vi "FRIC_navX_Internal_Serial_ProcessingLoop.vi"(7 "Device Number":T3, 11 "Rate (4Hz-200Hz)":u8=50 min=4 max=200) -> ()   [LabVIEW 2016, in "navX Library.lvlib"]
doc: "This navX VI handles the reading/writing for the navX. All of the good stuff is in here.\nTHIS VI SHOULD NOT BE CALLED BY THE USER!"
uses:
  navX Library.lvlib
  _TypeDefs/Z900_navX_SerialStreamTypeDef.ctl
  _TypeDefs/FRIC_navX_DeviceNumbersTypeDef.ctl
  <vilib>/Rock Robotics/WPI/SerialPort/WPI_SerialPort.ctl
  _TypeDefs/FRIC_navX_I2C Process Loop TypeDef.ctl
  _TypeDefs/FRIC_navX_ProcessingLoopStatesTypeDef_I2C.ctl
  _TypeDefs/Z900_navX_DeviceTypeDef.ctl
  _TypeDefs/Z900_navX_ProtocolTypeDef.ctl
  _TypeDefs/Z900_navX_NotifyPacketTypeDef.ctl
  _TypeDefs/Z900_navX_ActionTypeDef.ctl
  <vilib>/Rock Robotics/SystemInterfaces/i2clib/i2c_bus.ctl
  _TypeDefs/Z900_navX_IntegrationControlRegisters.ctl
  <vilib>/Rock Robotics/WPI/SPI/WPI_SPIDevRef.ctl
  <vilib>/Rock Robotics/SystemInterfaces/spilib/spi_bus.ctl
  <vilib>/Rock Robotics/WPI/SerialPort/WPI_SerialPortRef.ctl
  <vilib>/Platform/TimedLoop/XDataNode/timing_clust.ctl
  <vilib>/Platform/TimedLoop/XDataNode/nitl_modes.ctl
  <vilib>/Platform/TimedLoop/XDataNode/wakeup.ctl
  <vilib>/Rock Robotics/SystemInterfaces/Utilities/FPGA_UtilitiesRead LocalTime.vi
  <vilib>/Platform/TimedLoop/XDataNode/XDataNode.xnode
  <vilib>/Platform/TimedLoop/XDataNode/XDNodeRunTimeDep.lvlib
panel:
  in  "Tab Control":enum32{"Page 1", "Page 2"}(tab)
  in  "Halt":bool
  out "Connected":bool
  out "error":errorcluster
  in  "Stream Type":T1=enum."AHRSAndPositioning"
  in  "Serial Port":T2=enum."MXP TTL"
  out "Loop Time":i64
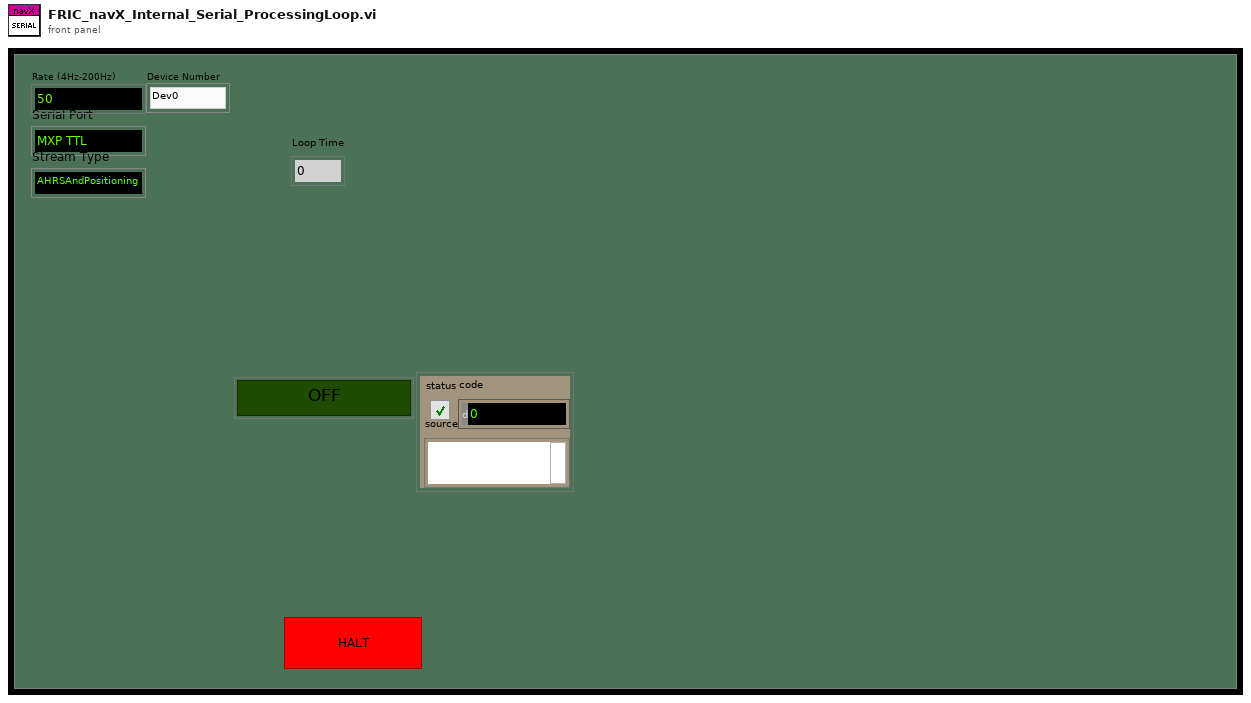
[diagram p1: front panel]
types:
  T1 = typedef "navX Library.lvlib/Z900_navX_SerialStreamTypeDef.ctl" = enum16{"YRPH", "Quaterinons", "Gyro/Raw", "AHRS", "AHRSAndPositioning", "AHRSAndPOSTime"}
  T2 = typedef "WPI_SerialPort.ctl" = enum16{"Onboard RS-232", "MXP TTL", "USB 1", "USB 2"}
  T3 = typedef "navX Library.lvlib/FRIC_navX_DeviceNumbersTypeDef.ctl" = enum16{"Dev0", "Dev1", "Dev2", "Dev3"}
  T4 = typedef "navX Library.lvlib/FRIC_navX_I2C Process Loop TypeDef.ctl" = cluster{"State Array":T5[], "error":errorcluster, "FPGA Cluster":cluster{"Last Valid FPGA Time":dbl, "Error Count":i32, "Initialized":bool}, "Device Info":T6, "I2CDevRef":cluster{"DevStatus":errorcluster, "Device Address":u8, "Handle":i32, "I2C Bus":T8}, "Registry":u8[], "Command Array":T9[], "Connected?":bool, "navX Device Memory Size":i32, "notification":T10, "Memory Size Set":bool, "SPIDevRef":T12, "navX Serial Open":cluster{"Stream Type":T1, "Serial Port":T2}, "SerialPortRef":T14, "Serial Read Buffer":string, "Serial Write Buffer":string[], "Device Number":T3, "navX SPI Open":cluster{"SPI Bus":T13, "Clock Rate (Hz)":dbl}, "Loop dt":i64, "current time":timestamp, "Loop Time":i64}
  T5 = typedef "navX Library.lvlib/FRIC_navX_ProcessingLoopStatesTypeDef_I2C.ctl" = enum16{"Process", "INI", "Check Packets Valid", "Close", "Clear VISA", "Generate Command", "Last Packet Valid", "Open", "Read", "Reset Serial", "Set Termination Char", "Update AE", "Wait", "Write", "Exit"}
  T6 = typedef "navX Library.lvlib/Z900_navX_DeviceTypeDef.ctl" = cluster{"Interface":cluster{"Protocol":T7, "Update Rate (4Hz-200Hz)":u8, "navX Open TypeDef":variant}, "Notify Packet":refnum<notifier>, "Loop VI Refnum":refnum<vi>, "Ready to Close Occurrence Refnum":refnum<k4>, "Name":string}
  T7 = typedef "navX Library.lvlib/Z900_navX_ProtocolTypeDef.ctl" = enum16{"SERIAL", "I2C", "SPI"}
  T8 = typedef "i2c_bus.ctl" = enum16{"I2C On-Board", "I2C MXP", "Invalid"}
  T9 = typedef "navX Library.lvlib/Z900_navX_IntegrationControlRegisters.ctl" = u8
  T10 = typedef "navX Library.lvlib/Z900_navX_NotifyPacketTypeDef.ctl" = cluster{"navX Action":T11, "Data":variant, "Stream Type":T1, "Device Number":T3}
  T11 = typedef "navX Library.lvlib/Z900_navX_ActionTypeDef.ctl" = enum16{"None", "Halt", "Normal Read", "Update Serial Protocol", "Update Rate Htz", "Zero-Yaw", "Zero-Displacement", "Zero-Velocity"}
  T12 = typedef "WPI_SPIDevRef.ctl" = cluster{"DevStatus":errorcluster, "Handle":i32, "SPI Bus":T13}
  T13 = typedef "spi_bus.ctl" = enum16{"SPI On-Board, CS0", "SPI On-Board, CS1", "SPI On-Board, CS2", "SPI On-Board, CS3", "SPI MXP", "Invalid"}
  T14 = typedef "WPI_SerialPortRef.ctl" = cluster{"DevStatus":errorcluster, "Serial Port Name":refnum<visa-resource-name>}
  T15 = typedef "XDNodeRunTimeDep.lvlib/timing_clust.ctl" = cluster{"Expected End [f-1]":u64, "Actual End [f-1]":u64, "Finished Late? [f-1]":bool, "Expected End [i-1]":u64, "Actual End [i-1]":u64, "Finished Late? [i-1]":bool, "Expected Start [i]":u64, "Actual Start [i]":u64, "Expected Start [f]":u64, "Actual Start [f]":u64, "Source Name":string, "Structure Name":string, "Period":i64, "Deadline":i64, "Offset":i64, "Start":i64, "Priority":i32, "Timeout":i32, "Mode":T16, "Wakeup Reason":T17, "Error":errorcluster, "Source Type":string, "Secondary Source Type":string, "Global End Time":u64, "Global Start Time":u64, "Frame Duration":u64, "Iteration Duration":u64, "Assigned CPU":i32, "I/O Scan Engine Mode":u32}
  T16 = typedef "XDNodeRunTimeDep.lvlib/nitl_modes.ctl" = enum32{"No Change", "Process missed periods, maintain original phase", "Discard missed periods, maintain original phase", "Process missed periods, ignore original phase", "Discard missed periods, ignore original phase"}
  T17 = typedef "XDNodeRunTimeDep.lvlib/wakeup.ctl" = enum32{"Normal", "Aborted", "Asynchronous wakeup", "Timing source error", "Timed loop error", "Timeout"}
  T18 = cluster{"Last Valid FPGA Time":dbl, "Error Count":i32, "Initialized":bool}
  T19 = typedef "Z900_navX_NotifyPacketTypeDef.ctl" = cluster{"navX Action":T20, "Data":variant, "Stream Type":T21, "Device Number":T22}
  T20 = typedef "Z900_navX_ActionTypeDef.ctl" = enum16{"None", "Halt", "Normal Read", "Update Serial Protocol", "Update Rate Htz", "Zero-Yaw", "Zero-Displacement", "Zero-Velocity"}
  T21 = typedef "Z900_navX_SerialStreamTypeDef.ctl" = enum16{"YRPH", "Quaterinons", "Gyro/Raw", "AHRS", "AHRSAndPositioning", "AHRSAndPOSTime"}
  T22 = typedef "FRIC_navX_DeviceNumbersTypeDef.ctl" = enum16{"Dev0", "Dev1", "Dev2", "Dev3"}
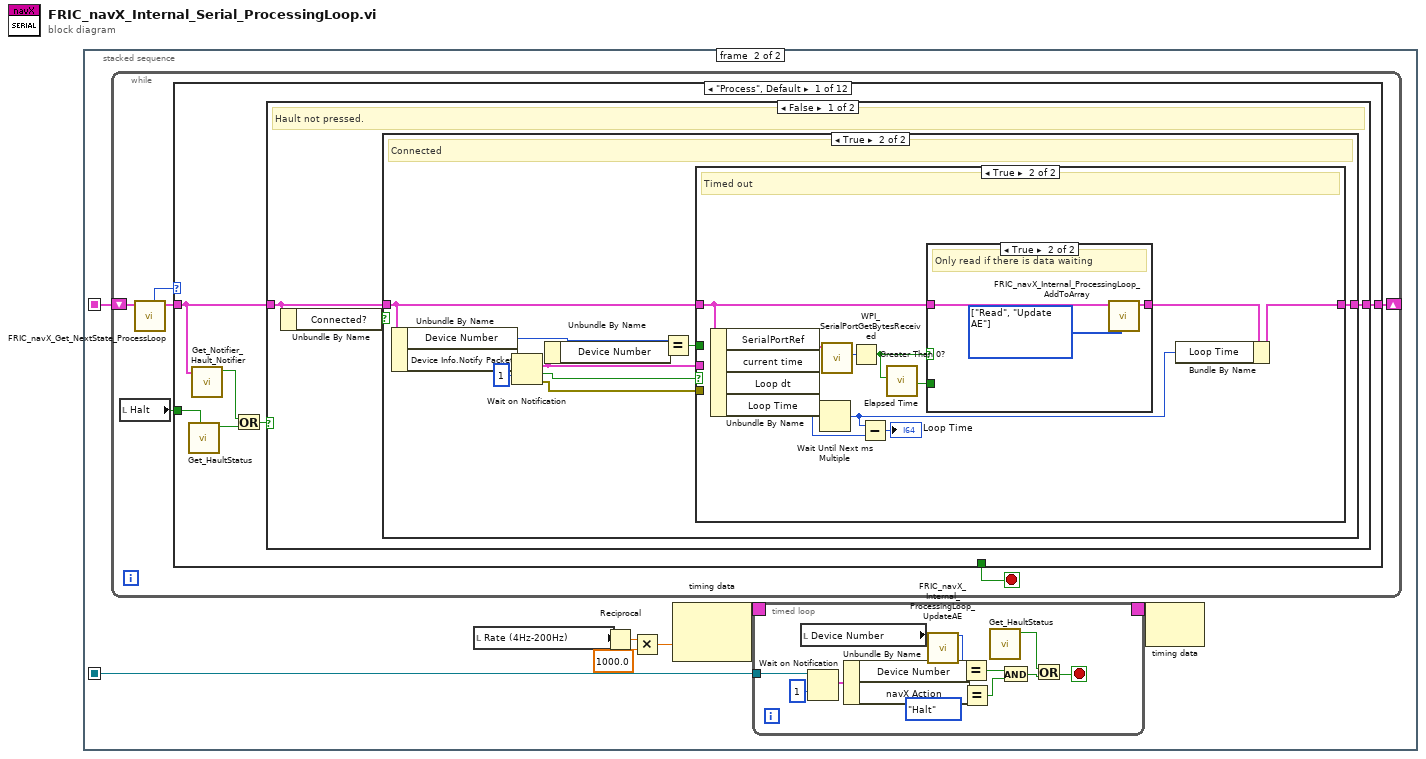
[diagram p0: block diagram]
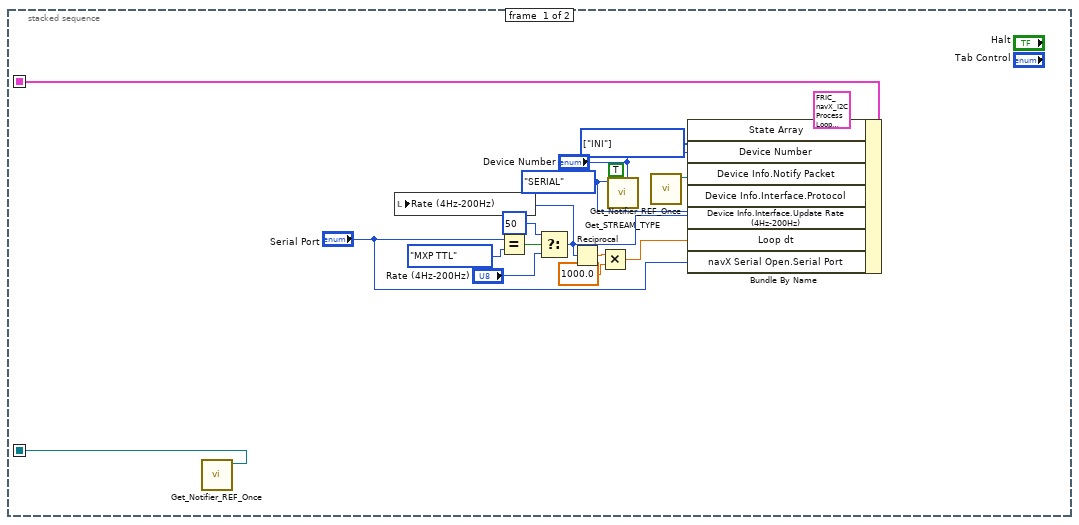
[diagram p2: hidden frame]
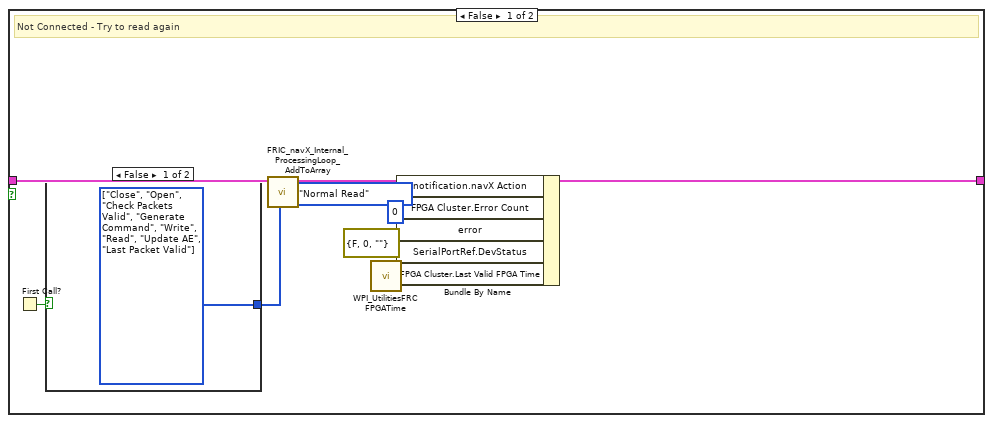
[diagram p3: hidden frame]
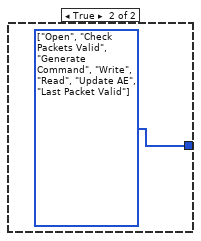
[diagram p4: hidden frame]
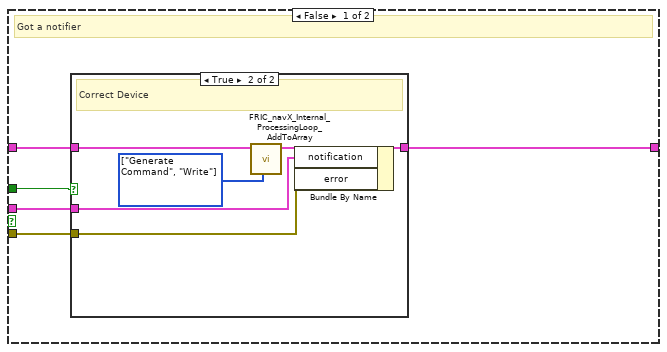
[diagram p5: hidden frame]
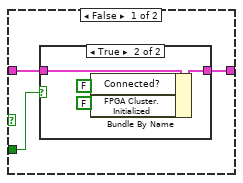
[diagram p7: hidden frame]
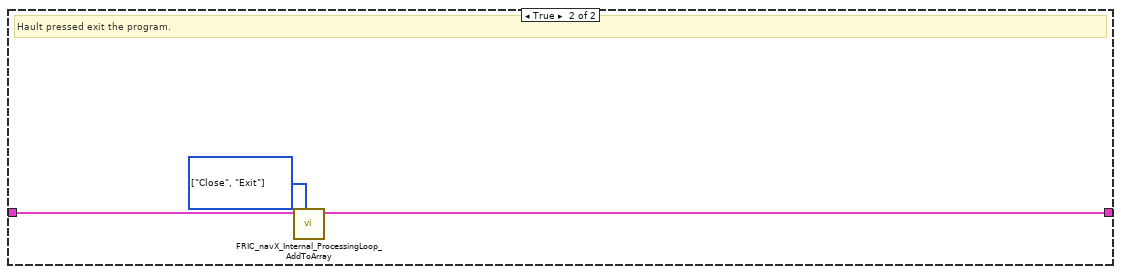
[diagram p9: hidden frame]
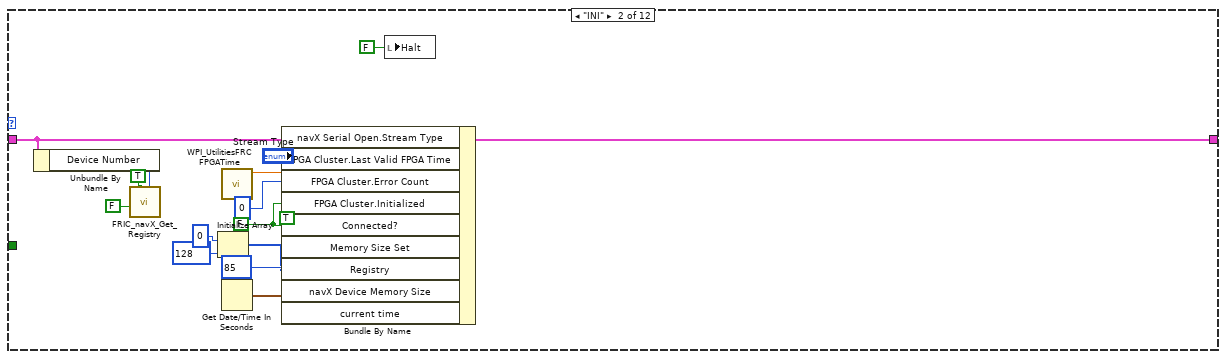
[diagram p10: hidden frame]
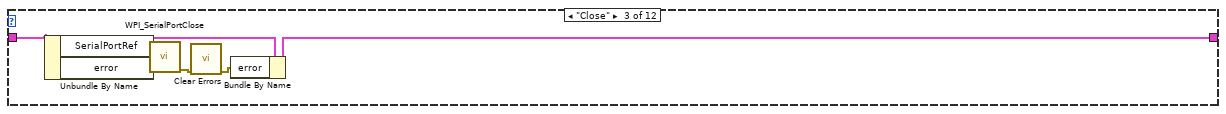
[diagram p11: hidden frame]
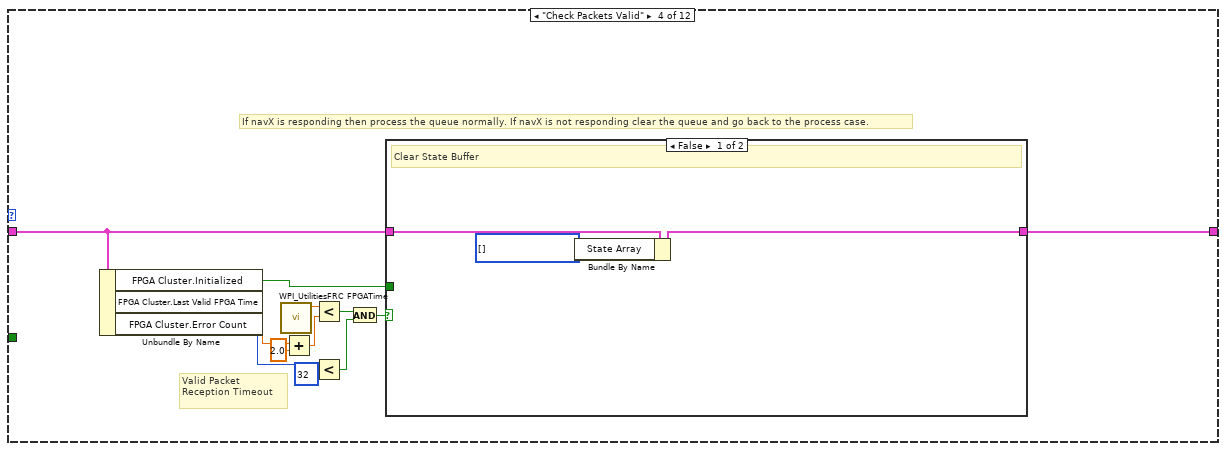
[diagram p12: hidden frame]
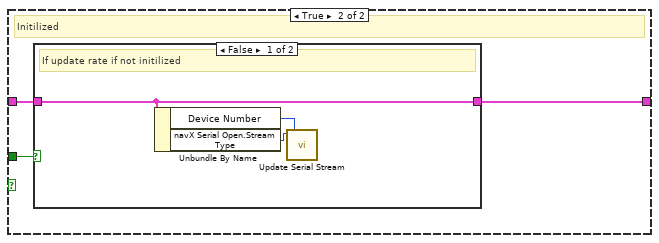
[diagram p13: hidden frame]
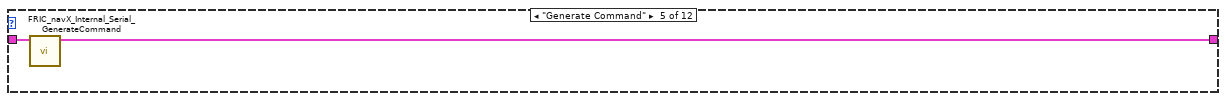
[diagram p15: hidden frame]
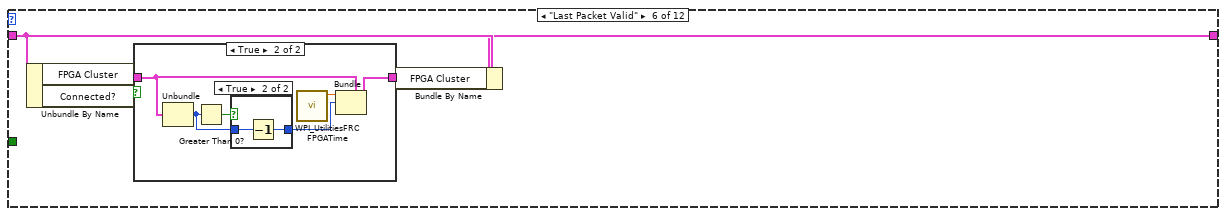
[diagram p16: hidden frame]
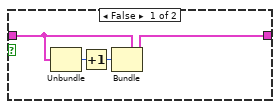
[diagram p17: hidden frame]
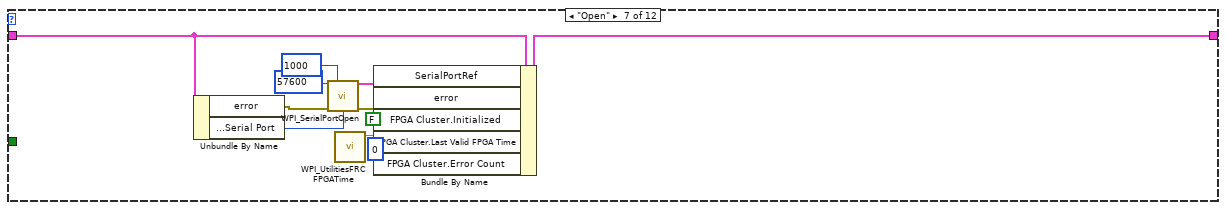
[diagram p19: hidden frame]
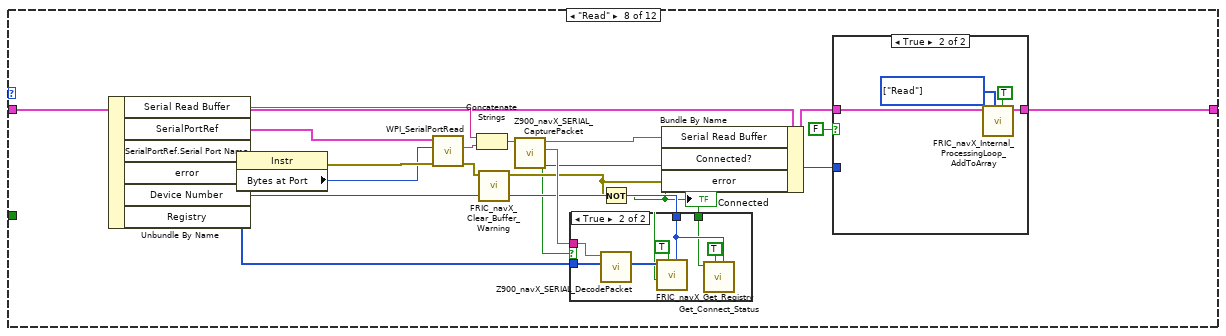
[diagram p20: hidden frame]
diagram:
  n1 = stacked-sequence {
    seq-local: [w17 _] -> [_ w25]
    seq-local: [w13 _] -> [_ w18]
    frame #0 {
      w1 = Z900_navX_ProtocolTypeDef."SERIAL" ("Protocol")
      w15 = T5[] [enum."INI"] items=["Process", "INI", "Check Packets Valid", "Close", "Clear VISA", "Generate Command", "Last Packet Valid", "Open", "Read", "Reset Serial", "Set Termination Char", "Update AE", "Wait", "Write", "Exit"] ("State Array")
      n2 = call "Get_Notifier_REF_Once.vi"() -> ("notifier ref out"=w13:refnum<notifier>)  [unwired: 10 in, 1 out]
      n3 = Equal?(x="Serial Port", y=WPI_SerialPort."MXP TTL") -> (x = y?=w11:bool)
      n4 = Select(t=u8 50, s=w11, f="Rate (4Hz-200Hz)") -> (s? t:f=w6:u8)
      n5 = local write "Rate (4Hz-200Hz)"(w6) -> ()
      n6 = Reciprocal(x=w6) -> (1/x=w9:dbl)
      n7 = Multiply(x=w9, y=1000.0) -> (x*y=w7:dbl)
      n8 = call "Get_STREAM_TYPE.vi"("Device Number"="Device Number", "Update"=TRUE, "Protocol (in)"=w1) -> ()  [unwired: 8 in, 1 out]
      n9 = call "Get_Notifier_REF_Once.vi"() -> ("notifier ref out"=w14:refnum<notifier>)  [unwired: 10 in, 1 out]
      n10 = Bundle By Name(cluster=T4 {"State Array"=[enum."INI", enum."Open"], "error"={"status"=FALSE, "code"=0, "source"=""}, "FPGA Cluster"={"Last Valid FPGA Time"=0.0, "Error Count"=0, "Initialized"=FALSE}, "Device Info"={"Interface"={"Protocol"=enum."SERIAL", "Update Rate (4Hz-200Hz)"=4, "navX Open TypeDef"=variant}, "Notify Packet"=refnum, "Loop VI Refnum"=refnum, "Ready to Close Occurrence Refnum"=refnum, "Name"=""}, "I2CDevRef"={"DevStatus"={"status"=FALSE, "code"=0, "source"=""}, "Device Address"=0, "Handle"=0, "I2C Bus"=enum."Invalid"}, "Registry"=[], "Command Array"=[214, 32], "Connected?"=FALSE, "navX Device Memory Size"=85, "notification"={"navX Action"=enum."None", "Data"=variant, "Stream Type"=enum."YRPH", "Device Number"=enum."Dev0"}, "Memory Size Set"=FALSE, "SPIDevRef"={"DevStatus"={"status"=FALSE, "code"=0, "source"=""}, "Handle"=0, "SPI Bus"=enum."SPI On-Board, CS0"}, "navX Serial Open"={"Stream Type"=enum."YRPH", "Serial Port"=enum."Onboard RS-232"}, "SerialPortRef"={"DevStatus"={"status"=FALSE, "code"=0, "source"=""}, "Serial Port Name"=""}, "Serial Read Buffer"="", "Serial Write Buffer"=[], "Device Number"=enum."Dev0", "navX SPI Open"={"SPI Bus"=enum."SPI MXP", "Clock Rate (Hz)"=500000.0}, "Loop dt"=0, "current time"=timestamp(0 s since 1904-01-01), "Loop Time"=0} ("I2C Process Loop TypeDef"), "State Array"=w15, "Device Number"="Device Number", "Device Info.Notify Packet"=w14, "Device Info.Interface.Protocol"=w1, "Device Info.Interface.Update Rate (4Hz-200Hz)"=w6, "Loop dt"=w7, "navX Serial Open.Serial Port"="Serial Port") -> (w17:T4)
    }
    frame #1 {
      n11 = while {
        shift-right: [w45] -> _
        shift-left: w25 -> [w48]
        stop <- w49 stop-if-true
        n12 = local read "Halt"() -> (w44:bool)
        n13 = call "FRIC_navX_Get_NextState_ProcessLoop.vi"("I2C Process Loop TypeDef (in)"=w48) -> ("I2C Process Loop TypeDef (out)"=w47:T4, "Current State"=w46:T5)  [unwired: 9 in]
        n14 = case shown="\"Process\", Default" w46 {
          tunnel: [_ _ _ _ _ _ _ _ _ _ TRUE _] -> w49
          tunnel: w47 -> [w53 w121 w138 w142 w162 w166 w191 w202 w229 w242 w249 w257]
          tunnel: [w55 w128 w137 w143 w161 w165 w190 w200 w230 w231 w249 w257] -> w45
          tunnel: w44 -> [w54 _ _ _ _ _ _ _ _ _ _ _]
          frame "Process", Default {
            n15 = call "Get_HaultStatus.vi"("Update"=w54) -> ("Hault"=w51:bool)  [unwired: 10 in]
            n16 = call "Get_Notifier_Hault_Notifier.vi"("Process Loop TypeDef (in)"=w53) -> ("Hault Notifier"=w52:bool)  [unwired: 10 in]
            n17 = Or(x=w52, y=w51) -> (x .or. y?=w50:bool)
            n18 = case shown="False" w50 {
              tunnel: [w58 w115] -> w55
              tunnel: w53 -> [w56 w116]
              frame False {
                # "Hault not pressed."
                n19 = Unbundle By Name(w56) -> ("Connected?"=w57:bool)
                n20 = case shown="True" w57 {
                  tunnel: w56 -> [w67 w78]
                  tunnel: [w64 w79] -> w58
                  frame False {
                    w60 = errorcluster {"status"=FALSE, "code"=0, "source"=""} ("error")
                    # "Not Connected - Try to read again"
                    n21 = First Call?() -> (First Call?: T/F=w61:bool)
                    n22 = case shown="False" w61 {
                      tunnel: [w68 w69] -> w66
                      frame False {
                        w68 = T5[] [enum."Close", enum."Open", enum."Check Packets Valid", enum."Generate Command", enum."Write", enum."Read", enum."Update AE", enum."Last Packet Valid"] items=["Process", "INI", "Check Packets Valid", "Close", "Clear VISA", "Generate Command", "Last Packet Valid", "Open", "Read", "Reset Serial", "Set Termination Char", "Update AE", "Wait", "Write", "Exit"]
                      }
                      frame True {
                        w69 = T5[] [enum."Open", enum."Check Packets Valid", enum."Generate Command", enum."Write", enum."Read", enum."Update AE", enum."Last Packet Valid"] items=["Process", "INI", "Check Packets Valid", "Close", "Clear VISA", "Generate Command", "Last Packet Valid", "Open", "Read", "Reset Serial", "Set Termination Char", "Update AE", "Wait", "Write", "Exit"]
                      }
                    }
                    n23 = call "FRIC_navX_Internal_ProcessingLoop_AddToArray.vi"("States Array"=w66, "I2C Process Loop TypeDef (in)"=w67) -> ("I2C Process Loop TypeDef (out)"=w65:T4)  [unwired: 9 in]
                    n24 = call <vilib>:"WPI_UtilitiesFRC FPGATime.vi"() -> ("FPGA Time"=w59:dbl)  [unwired: 10 in, 1 out]
                    n25 = Bundle By Name(cluster=w65, "notification.navX Action"=Z900_navX_ActionTypeDef."Normal Read", "FPGA Cluster.Error Count"=0, "error"=w60, "SerialPortRef.DevStatus"=w60, "FPGA Cluster.Last Valid FPGA Time"=w59) -> (w64:T4)
                  }
                  frame True {
                    # "Connected"
                    n26 = Unbundle By Name(w78) -> ("Device Number"=w72:T3, "Device Info.Notify Packet"=w77:refnum<notifier>)
                    n27 = Wait on Notification(notifier=w77, timeout in ms (-1)=1) -> (notification=w73:T10, timed out?=w74:bool, error out=w75:errorcluster)  [unwired: 2 in, 1 out]
                    n28 = Unbundle By Name(w73) -> ("Device Number"=w71:T3)
                    n29 = Equal?(x=w72, y=w71) -> (x = y?=w70:bool)
                    n30 = case shown="True" w74 {
                      tunnel: w78 -> [w84 w99]
                      tunnel: [w83 w96] -> w79
                      tunnel: w73 -> [w82 _]
                      tunnel: w75 -> [w81 _]
                      tunnel: w70 -> [w80 _]
                      frame False {
                        # "Got a notifier"
                        n31 = case shown="True" w80 {
                          tunnel: w84 -> [w85 w91]
                          tunnel: [w85 w90] -> w83
                          tunnel: w82 -> [_ w89]
                          tunnel: w81 -> [_ w86]
                          frame False {
                          }
                          frame True {
                            w87 = T5[] [enum."Generate Command", enum."Write"] items=["Process", "INI", "Check Packets Valid", "Close", "Clear VISA", "Generate Command", "Last Packet Valid", "Open", "Read", "Reset Serial", "Set Termination Char", "Update AE", "Wait", "Write", "Exit"] ("States Array")
                            # "Correct Device"
                            n32 = call "FRIC_navX_Internal_ProcessingLoop_AddToArray.vi"("States Array"=w87, "I2C Process Loop TypeDef (in)"=w91) -> ("I2C Process Loop TypeDef (out)"=w88:T4)  [unwired: 9 in]
                            n33 = Bundle By Name(cluster=w88, "notification"=w89, "error"=w86) -> (w90:T4)
                          }
                        }
                      }
                      frame True {
                        # "Timed out"
                        n34 = Unbundle By Name(w99) -> ("SerialPortRef"=w101:T14, "Loop dt"=w95:i64, "Loop Time"=w93:i64)  [unwired: 1 out]
                        n35 = Wait Until Next ms Multiple(millisecond multiple=w95) -> (millisecond timer value=w94:u32)
                        n36 = call <vilib>:"WPI_SerialPortGetBytesReceived.vi"("SerialPortRef"=w101) -> ("Bytes at Port"=w100:u32)  [unwired: 8 in, 2 out]
                        n37 = Greater Than 0?(x=w100) -> (x > 0?=w98:bool)
                        n38 = Subtract(x=w94, y=w93) -> (x-y=→"Loop Time":i64)
                        n39 = call "Elapsed Time"("Reset"=w98) -> ("Time has Elapsed"=w97:bool)  [unwired: 11 in, 7 out]
                        n40 = case shown="True" w98 {
                          tunnel: [w103 w112] -> w102
                          tunnel: w99 -> [w104 w111]
                          tunnel: w97 -> [w105 _]
                          frame False {
                            n41 = case shown="True" w105 {
                              tunnel: w104 -> [w106 w110]
                              tunnel: [w106 w109] -> w103
                              frame False {
                              }
                              frame True {
                                n42 = Bundle By Name(cluster=w110, "Connected?"=FALSE, "FPGA Cluster.Initialized"=FALSE) -> (w109:T4)
                              }
                            }
                          }
                          frame True {
                            w113 = T5[] [enum."Read", enum."Update AE"] items=["Process", "INI", "Check Packets Valid", "Close", "Clear VISA", "Generate Command", "Last Packet Valid", "Open", "Read", "Reset Serial", "Set Termination Char", "Update AE", "Wait", "Write", "Exit"]
                            # "Only read if there is data waiting"
                            n43 = call "FRIC_navX_Internal_ProcessingLoop_AddToArray.vi"("States Array"=w113, "I2C Process Loop TypeDef (in)"=w111) -> ("I2C Process Loop TypeDef (out)"=w112:T4)  [unwired: 9 in]
                          }
                        }
                        n44 = Bundle By Name(cluster=w102, "Loop Time"=w94) -> (w96:T4)
                      }
                    }
                  }
                }
              }
              frame True {
                w114 = T5[] [enum."Close", enum."Exit"] items=["Process", "INI", "Check Packets Valid", "Close", "Clear VISA", "Generate Command", "Last Packet Valid", "Open", "Read", "Reset Serial", "Set Termination Char", "Update AE", "Wait", "Write", "Exit"] ("States Array")
                # "Hault pressed exit the program."
                n45 = call "FRIC_navX_Internal_ProcessingLoop_AddToArray.vi"("States Array"=w114, "I2C Process Loop TypeDef (in)"=w116) -> ("I2C Process Loop TypeDef (out)"=w115:T4)  [unwired: 9 in]
              }
            }
          }
          frame "INI" {
            w126 = FALSE ("Initialized")
            n46 = Unbundle By Name(w121) -> ("Device Number"=w120:T3)
            n47 = call "FRIC_navX_Get_Registry.vi"("Device Number"=w120, "Update"=TRUE, "Connected?"=FALSE) -> ()  [unwired: 7 in, 2 out]
            n48 = Initialize Array(u8 0 ("Received Data"), 128 ("hex")) -> (w124:u8[])
            n49 = call <vilib>:"WPI_UtilitiesFRC FPGATime.vi"() -> ("FPGA Time"=w130:dbl)  [unwired: 10 in, 1 out]
            n50 = Get Date/Time In Seconds() -> (seconds since 1Jan1904=w117:timestamp)
            n51 = Bundle By Name(cluster=w121, "navX Serial Open.Stream Type"="Stream Type", "FPGA Cluster.Last Valid FPGA Time"=w130, "FPGA Cluster.Error Count"=0 ("Error Count"), "FPGA Cluster.Initialized"=w126, "Connected?"=w126, "Memory Size Set"=TRUE, "Registry"=w124, "navX Device Memory Size"=85 ("hex"), "current time"=w117) -> (w128:T4)
            n52 = local write "Halt"(FALSE ("Halt")) -> ()
          }
          frame "Close" {
            n53 = Unbundle By Name(w138) -> ("SerialPortRef"=w135:T14, "error"=w134:errorcluster)
            n54 = call <vilib>:"WPI_SerialPortClose.vi"("error in (no error)"=w134, "SerialPortRef"=w135) -> ("error out"=w133:errorcluster)  [unwired: 9 in]
            n55 = call <vilib>:"Clear Errors.vi"("error in (no error)"=w133) -> ("error out"=w136:errorcluster)  [unwired: 5 in, 1 out]
            n56 = Bundle By Name(cluster=w138, "error"=w136) -> (w137:T4)
          }
          frame "Check Packets Valid" {
            # "If navX is responding then process the queue normally. If navX is not responding clear the queue and go back to the process case."
            # "Valid Packet Reception Timeout"
            n57 = Unbundle By Name(w142) -> ("FPGA Cluster.Initialized"=w140:bool, "FPGA Cluster.Last Valid FPGA Time"=w141:dbl, "FPGA Cluster.Error Count"=w139:i32)
            n58 = call <vilib>:"WPI_UtilitiesFRC FPGATime.vi"() -> ("FPGA Time"=w148:dbl)  [unwired: 10 in, 1 out]
            n59 = Add(x=w141, y=2.0) -> (x+y=w149:dbl)
            n60 = Less?(x=w148, y=w149) -> (x < y?=w146:bool)
            n61 = Less?(x=w139, y=32) -> (x < y?=w145:bool)
            n62 = And(x=w146, y=w145) -> (x .and. y?=w144:bool)
            n63 = case shown="False" w144 {
              tunnel: w142 -> [w153 w156]
              tunnel: [w152 w155] -> w143
              tunnel: w140 -> [_ w154]
              frame False {
                w151 = T5[] [] items=["Process", "INI", "Check Packets Valid", "Close", "Clear VISA", "Generate Command", "Last Packet Valid", "Open", "Read", "Reset Serial", "Set Termination Char", "Update AE", "Wait", "Write", "Exit"] ("f")
                # "Clear State Buffer"
                n64 = Bundle By Name(cluster=w153, "State Array"=w151) -> (w152:T4)
              }
              frame True {
                # "Initilized"
                n65 = case shown="False" w154 {
                  tunnel: w156 -> [w159 w160]
                  tunnel: [w159 w160] -> w155
                  frame False {
                    # "If update rate if not initilized"
                    n66 = Unbundle By Name(w159) -> ("Device Number"=w158:T3, "navX Serial Open.Stream Type"=w157:T1)
                    n67 = call "Update Serial Stream.vi"("Device Number"=w158, "Stream Type"=w157) -> ()  [unwired: 10 in]
                  }
                  frame True {
                    # "Everything is good keep going"
                  }
                }
              }
            }
          }
          frame "Generate Command" {
            n68 = call "FRIC_navX_Internal_Serial_GenerateCommand.vi"("Serial Process Loop TypeDef (in)"=w162) -> ("Serial Process Loop TypeDef (out)"=w161:T4)  [unwired: 10 in]
          }
          frame "Last Packet Valid" {
            n69 = Unbundle By Name(w166) -> ("FPGA Cluster"=w167:T18, "Connected?"=w163:bool)
            n70 = case shown="True" w163 {
              tunnel: [w170 w177] -> w164
              tunnel: w167 -> [w169 w173]
              frame False {
                n71 = Unbundle(w169) -> ("Error Count"=w168:i32)  [unwired: 2 out]
                n72 = Increment(x=w168) -> (x+1=w171:i32)
                n73 = Bundle(cluster=w169, "Error Count"=w171) -> (w170:T18)  [unwired: 2 in]
              }
              frame True {
                n74 = Unbundle(w173) -> ("Error Count"=w172:i32)  [unwired: 2 out]
                n75 = Greater Than 0?(x=w172) -> (x > 0?=w175:bool)
                n76 = case shown="True" w175 {
                  tunnel: [w178 w180] -> w174
                  tunnel: w172 -> [w178 w179]
                  frame False {
                  }
                  frame True {
                    n77 = Decrement(x=w179) -> (x-1=w180:i32)
                  }
                }
                n78 = call <vilib>:"WPI_UtilitiesFRC FPGATime.vi"() -> ("FPGA Time"=w176:dbl)  [unwired: 10 in, 1 out]
                n79 = Bundle(cluster=w173, "Last Valid FPGA Time"=w176, "Error Count"=w174) -> (w177:T18)  [unwired: 1 in]
              }
            }
            n80 = Bundle By Name(cluster=w166, "FPGA Cluster"=w164) -> (w165:T4)
          }
          frame "Open" {
            n81 = Unbundle By Name(w191) -> ("error"=w182:errorcluster, "navX Serial Open.Serial Port"=w181:T2)
            n82 = call <vilib>:"WPI_SerialPortOpen.vi"("Baud Rate"=u32 57600, "Timeout Value (ms)"=u32 1000, "error in (no error)"=w182, "Serial Port"=w181) -> ("SerialPortRef"=w185:T14, "error out"=w186:errorcluster)  [unwired: 10 in]
            n83 = call <vilib>:"WPI_UtilitiesFRC FPGATime.vi"() -> ("FPGA Time"=w184:dbl)  [unwired: 10 in, 1 out]
            n84 = Bundle By Name(cluster=w191, "SerialPortRef"=w185, "error"=w186, "FPGA Cluster.Initialized"=FALSE ("Initialized"), "FPGA Cluster.Last Valid FPGA Time"=w184, "FPGA Cluster.Error Count"=0) -> (w190:T4)
          }
          frame "Read" {
            n85 = Unbundle By Name(w202) -> ("Serial Read Buffer"=w208:string, "SerialPortRef"=w209:T14, "SerialPortRef.Serial Port Name"=w212:refnum<visa-resource-name>, "error"=w211:errorcluster, "Device Number"=w199:T3, "Registry"=w204:u8[])
            n86 = property class="Instr"(reference=w212, error in=w211) -> (error out=w206:errorcluster, "Bytes at Port"=w193:u32)  [unwired: 1 in]
            n87 = call <vilib>:"WPI_SerialPortRead.vi"("error in (no error)"=w206, "Num Bytes to Read"=w193, "SerialPortRef"=w209) -> ("error out"=w196:errorcluster, "Buffer"=w210:string)  [unwired: 6 in, 1 out]
            n88 = Concatenate Strings(w208, w210) -> (w207:string)
            n89 = call "FRIC_navX_Clear_Buffer_Warning.vi"("error in"=w196) -> ("error out"=w195:errorcluster)  [unwired: 10 in]
            n90 = call "Z900_navX_SERIAL_CapturePacket.vi"("Buffer"=w207) -> ("Packet Size"=w197:i32, "Packet Located"=w194:bool, "Packet"=w203:string, "Buffer"=w205:string)  [unwired: 7 in]
            n91 = Not(x=w195) -> (.not. x?=w198:bool)
            "Connected" <- w198
            n92 = case shown="True" w194 {
              tunnel: w204 -> [_ w218]
              tunnel: w203 -> [_ w217]
              tunnel: w199 -> [_ w215]
              tunnel: w198 -> [_ w214]
              frame False {
              }
              frame True {
                n93 = call "Z900_navX_SERIAL_DecodePacket.vi"("Data (in)"=w218, "Packet (in)"=w217) -> ("Data"=w219:u8[])  [unwired: 7 in, 2 out]
                n94 = call "FRIC_navX_Get_Registry.vi"("Device Number"=w215, "Update"=TRUE, "Connected?"=w214, "Registry (in)"=w219) -> ()  [unwired: 6 in, 2 out]
                n95 = call "Get_Connect_Status.vi"("Device Number"=w215, "Update"=TRUE, "Connected"=w214) -> ()  [unwired: 8 in, 1 out]
              }
            }
            n96 = Bundle By Name(cluster=w202, "Serial Read Buffer"=w205, "Connected?"=w198, "error"=w195) -> (w201:T4)
            n97 = case shown="True" FALSE {
              tunnel: w201 -> [w220 w224]
              tunnel: [w220 w223] -> w200
              tunnel: w197 -> [_ _]
              frame False {
              }
              frame True {
                w222 = T5[] [enum."Read"] items=["Process", "INI", "Check Packets Valid", "Close", "Clear VISA", "Generate Command", "Last Packet Valid", "Open", "Read", "Reset Serial", "Set Termination Char", "Update AE", "Wait", "Write", "Exit"] ("States Array")
                n98 = call "FRIC_navX_Internal_ProcessingLoop_AddToArray.vi"("Add to beginning"=TRUE, "States Array"=w222, "I2C Process Loop TypeDef (in)"=w224) -> ("I2C Process Loop TypeDef (out)"=w223:T4)  [unwired: 8 in]
              }
            }
          }
          frame "Reset Serial" {
            n99 = Unbundle By Name(w229) -> ("SerialPortRef"=w228:T14, "error"=w226:errorcluster)
            n100 = call <vilib>:"WPI_SerialPortReset.vi"("error in (no error)"=w226, "SerialPortRef"=w228) -> ("error out"=w225:errorcluster, "SerialPortRef"=w227:T14)  [unwired: 8 in]
            n101 = Bundle By Name(cluster=w229, "SerialPortRef"=w227, "error"=w225) -> (w230:T4)
          }
          frame "Write" {
            n102 = Unbundle By Name(w242) -> ("SerialPortRef"=w240:T14, "Serial Write Buffer"=w237:string[], "SerialPortRef.DevStatus"=w241:errorcluster)
            n103 = Delete From Array(array=w237, index=0) -> (deleted portion=w236:string, array with subset deleted=w233:string[])  [unwired: 1 in]
            n104 = call <vilib>:"WPI_SerialPortWrite.vi"("error in (no error)"=w241, "Buffer"=w236, "SerialPortRef"=w240) -> ("error out"=w239:errorcluster, "SerialPortRef"=w238:T14)  [unwired: 6 in, 1 out]
            n105 = Empty Array?(array=w233) -> (empty?=w232:bool)
            n106 = Bundle By Name(cluster=w242, "SerialPortRef"=w238, "error"=w239, "Serial Write Buffer"=w233) -> (w234:T4)
            n107 = case shown="False" w232 {
              tunnel: [w246 w247] -> w231
              tunnel: w234 -> [w245 w247]
              frame False {
                w244 = T5[] [enum."Write"] items=["Process", "INI", "Check Packets Valid", "Close", "Clear VISA", "Generate Command", "Last Packet Valid", "Open", "Read", "Reset Serial", "Set Termination Char", "Update AE", "Wait", "Write", "Exit"] ("States Array")
                # "Write again because buffer is not empty."
                n108 = call "FRIC_navX_Internal_ProcessingLoop_AddToArray.vi"("Add to beginning"=TRUE, "States Array"=w244, "I2C Process Loop TypeDef (in)"=w245) -> ("I2C Process Loop TypeDef (out)"=w246:T4)  [unwired: 8 in]
              }
              frame True {
                # "Process the rest of the state array"
              }
            }
          }
          frame "Exit" {
            n109 = Unbundle By Name(w249) -> ("Device Info"=w248:T6)
            n110 = in-place {
              in-place-border: w248 -> [w252]
              # "Set Occurence of Close"
              n111 = Unbundle By Name(w252) -> ("Ready to Close Occurrence Refnum"=w253:refnum<k4>)
              n112 = local write "Halt"(FALSE ("Halt")) -> ()
              n113 = Set Occurrence(w253) -> ()
            }
          }
          frame "Update AE" {
            n114 = Unbundle By Name(w257) -> ("Device Number"=w255:T3, "error"=w256:errorcluster)
            "error" <- w256
            n115 = call "Get_Error_Status.vi"("Device Number"=w255, "Update"=TRUE, "error in"=w256) -> ()  [unwired: 8 in, 1 out]
          }
        }
      }
      n116 = local read "Rate (4Hz-200Hz)"() -> (w23:u8)
      n117 = Reciprocal(x=w23) -> (1/x=w22:dbl)
      n118 = Multiply(x=w22, y=1000.0) -> (x*y=w19:dbl)
      n119 = node-c288(w19) -> (w21:T15)  [unwired: 1 in]
      n120 = timed-loop {
        timing: w21 -> [_]
        timing-out: [_] -> w20
        tunnel: w18 -> [w29]
        stop <- w28 stop-if-true
        n121 = local read "Device Number"() -> (w32:T3)
        n122 = Wait on Notification(notifier=w29, timeout in ms (-1)=1) -> (notification=w34:T19)  [unwired: 2 in, 3 out]
        n123 = Unbundle By Name(w34) -> ("Device Number"=w33:T22, "navX Action"=w36:T20)
        n124 = call "FRIC_navX_Internal_ProcessingLoop_UpdateAE.vi"("Device Number"=w32) -> ()  [unwired: 15 in]
        n125 = Equal?(x=w32, y=w33) -> (x = y?=w31:bool)
        n126 = Equal?(x=w36, y=Z900_navX_ActionTypeDef."Halt") -> (x = y?=w30:bool)
        n127 = call "Get_HaultStatus.vi"() -> ("Hault"=w27:bool)  [unwired: 11 in]
        n128 = And(x=w31, y=w30) -> (x .and. y?=w26:bool)
        n129 = Or(x=w27, y=w26) -> (x .or. y?=w28:bool)
      }
      n130 = node-c288(w20) -> ()  [unwired: 1 out]
    }
  }
